vi "Load Setting.vi"(8 "error in":errorcluster, 11 "Class in":refnum<class>) -> (0 "error out":errorcluster, 3 "Class out":refnum<class>)   [LabVIEW 2023, in "Label-Driven UI.lvlib"]
doc: "어플리케이션 디렉토리/Config에서 저장된 값을 불러옵니다."
uses:
  Label-Driven UI.lvlib
  56708fb8-0744-4677-b418-acc78794b356.vi
  56708fb8-0744-4677-b418-acc78794b356.vi/a3a29cf6-1168-4dca-8b5f-a6d091da0069.vi
  Get VI Ref.vi
  Append Label to Error.vi
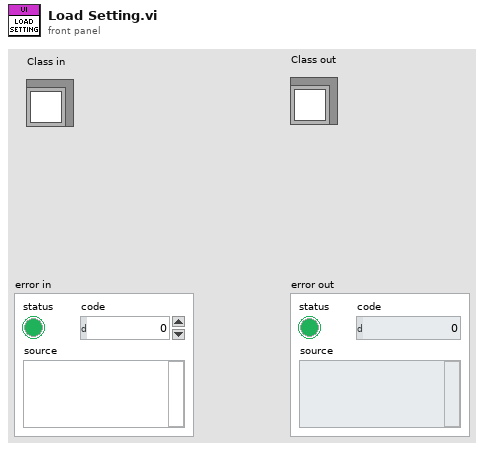
[diagram p1: front panel]
types:
  T1 = enum16{"big-endian, network order", "native, host order", "little-endian"}
  T2 = enum16{"open", "replace", "create", "open or create", "replace or create", "replace or create with confirmation"}
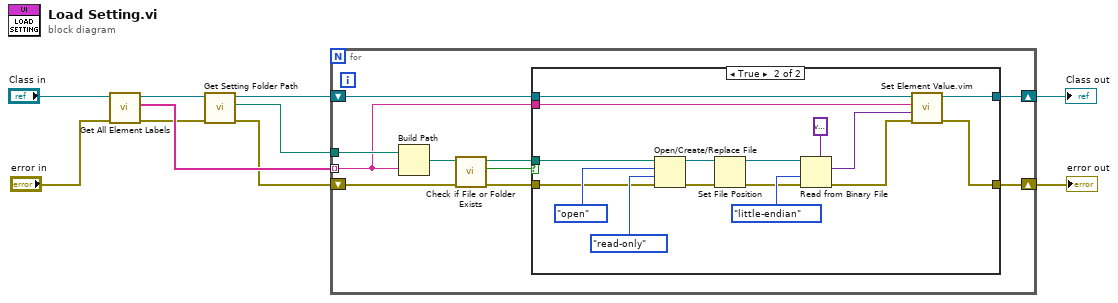
[diagram p0: block diagram]
diagram:
  n1 = call "Get All Element Labels.vi"("error in"="error in", "Class in"="Class in") -> ("error out"=w1:errorcluster, "Labels"=w9:string[], "Class out"=w8:refnum<class>)  [unwired: 7 in]
  n2 = call "Get Setting Folder Path.vi"("error in (no error)"=w1, "LabVIEW Object in"=w8) -> ("error out"=w5:errorcluster, "appended path"=w7:path, "LabVIEW Object out"=w6:refnum<class>)  [unwired: 7 in]
  n3 = for {
    tunnel: w9 -> [w15] mode=indexing
    tunnel: w7 -> [w18]
    shift-right: [w11] -> w4
    shift-left: w6 -> [w17]
    shift-right: [w12] -> w2
    shift-left: w5 -> [w13]
    n4 = Build Path(base path=w18, name or relative path=w15) -> (appended path=w20:path)
    n5 = call <vilib>:"Check if File or Folder Exists.vi"("error in (no error)"=w13, "path"=w20) -> ("error out"=w14:errorcluster, "file or folder exists?"=w19:bool, "dup path"=w16:path)  [unwired: 7 in]
    n6 = case shown="True" w19 {
      tunnel: w17 -> [w21 w27]
      tunnel: w16 -> [_ w33]
      tunnel: w15 -> [_ w26]
      tunnel: w14 -> [w22 w32]
      tunnel: [w22 w23] -> w12
      tunnel: [w21 w28] -> w11
      frame False {
      }
      frame True {
        n7 = Open/Create/Replace File(file path (use dialog)=w33, error in=w32, operation (0:open)=T2."open", access (0:read/write)=enum16{"read/write", "read-only", "write-only"}."read-only") -> (refnum out=w36:refnum<file>, error out=w30:errorcluster)  [unwired: 2 in, 1 out]
        n8 = Set File Position(refnum=w36, error in=w30) -> (refnum out=w31:refnum<file>, error out=w29:errorcluster)  [unwired: 2 in]
        n9 = Read from Binary File(5:variant, 8:w29, 9:T1."little-endian" ("byte order (0:big-endian, network order)"), 11:w31) -> (0:w24:errorcluster, 2:w25:variant)  [unwired: 2 in, 2 out]
        n10 = call "Set Element Value.vim"("error in"=w24, "Value"=w25, "Label"=w26, "Class in"=w27) -> ("error out"=w23:errorcluster, "Class out"=w28:refnum<class>)  [unwired: 6 in]
      }
    }
  }
  "Class out" <- w4
  "error out" <- w2
